vi "NewLeftSubpanel.vi"(8 "error in (no error)":errorcluster, 10 "NewPanel":i32, 11 "EmbeddedMainUI in":refnum<class "EmbeddedMainUI.lvclass">) -> (0 "error out":errorcluster, 3 "EmbeddedMainUI out":refnum<class "EmbeddedMainUI.lvclass">)   [LabVIEW 2016, in "EmbeddedMainUI.lvclass"]
uses:
  EmbeddedMainUI.lvclass
  <vilib>/Levylab/Embedded SMO UI/EmbeddedSMO.lvclass
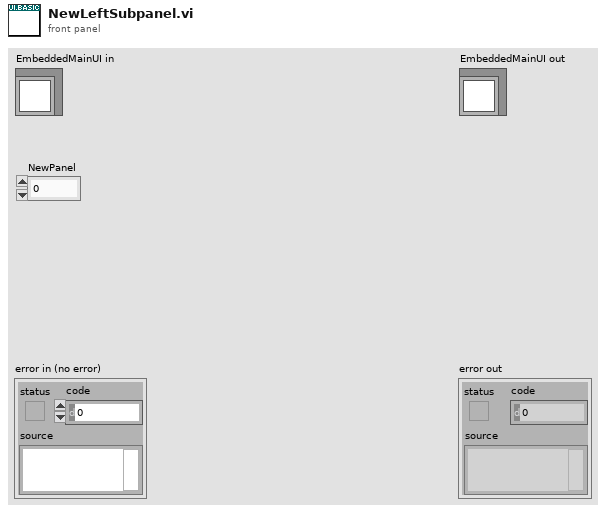
[diagram p1: front panel]
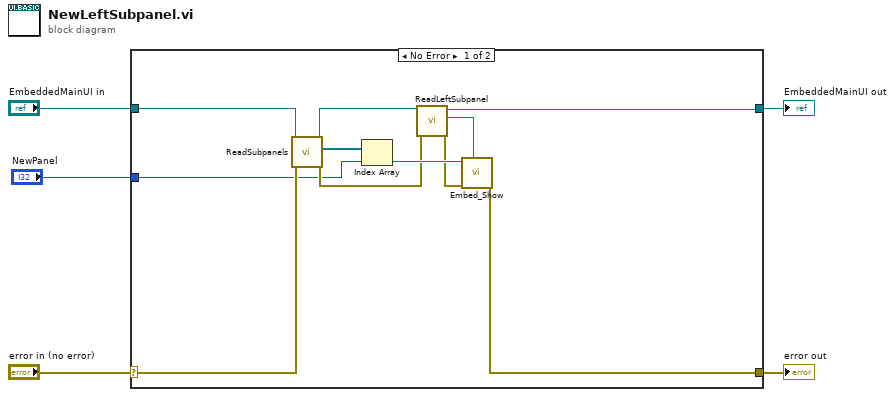
[diagram p0: block diagram]
diagram:
  n1 = case shown="No Error" "error in (no error)" {
    selector: "error in (no error)" -> [w8 w18]
    tunnel: [w7 w18] -> w4
    tunnel: [w11 w17] -> w2
    tunnel: "EmbeddedMainUI in" -> [w13 w17]
    tunnel: "NewPanel" -> [w6 _]
    frame No Error {
      n2 = call "ReadSubpanels.vi"("error in (no error)"=w8, "EmbeddedMainUI in"=w13) -> ("error out"=w10:errorcluster, "Subpanels"=w15:refnum<class "EmbeddedSMO.lvclass">[], "EmbeddedMainUI out"=w12:refnum<class "EmbeddedMainUI.lvclass">)  [unwired: 7 in]
      n3 = Index Array(array=w15, index=w6) -> (element=w16:refnum<class "EmbeddedSMO.lvclass">)
      n4 = call "ReadLeftSubpanel.vi"("error in (no error)"=w10, "EmbeddedMainUI in"=w12) -> ("error out"=w9:errorcluster, "Left Subpanel"=w14:refnum<vi>, "EmbeddedMainUI out"=w11:refnum<class "EmbeddedMainUI.lvclass">)  [unwired: 7 in]
      n5 = call <vilib>:"Embed_Show.vi"("Sub Panel"=w14, "error in (no error)"=w9, "EmbeddedSMO in"=w16) -> ("error out"=w7:errorcluster)  [unwired: 7 in, 1 out]
    }
    frame Error {
    }
  }
  "error out" <- w4
  "EmbeddedMainUI out" <- w2
